vi "Configure Trace.vi"(6 "Trace Unit (0: DBM)":i32(ring) items=["DBM", "W"], 7 "Enable Trace (T: Enable)":bool=TRUE, 8 "error in (no error)":errorcluster, 9 "Trace Duration (0.0001 s)":dbl=0.0001, 10 "Trace Delay (0 s)":dbl, 11 "VISA resource name":refnum<visa-resource-name>) -> (0 "error out":errorcluster, 3 "VISA resource name out":refnum<visa-resource-name>)   [LabVIEW 2014, in "Agilent U2000 Series.lvlib"]
doc: "Configures the measured power trace which includes:\nSpecifying the resolution type of trace to be captured.\nEnables/disables trace capture.\nSpecifying the trace units.\nSetting the duration of the trace and the delay between the delayed trigger point and the start of the trace.\n\nUsing this VI will set the sensor to normal mode. \n\nNotes:\nIn case of U2040 X-Series, it is applicable for U2042XA/U2044XA/U2049XA only."
uses:
  Agilent U2000 Series.lvlib
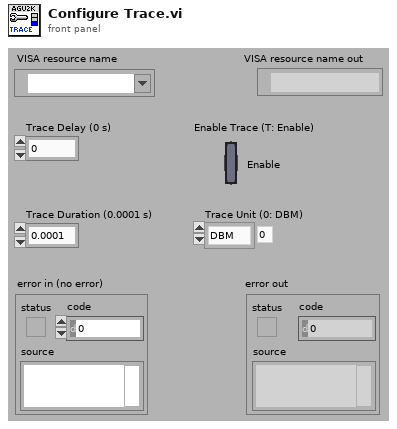
[diagram p1: front panel]
types:
  T1 = typedef "Agilent U2000 Series.lvlib/Extended User Data.ctl" = cluster{"U2000 Series Mode":u16, "Trigger Source Int/Ext":bool}
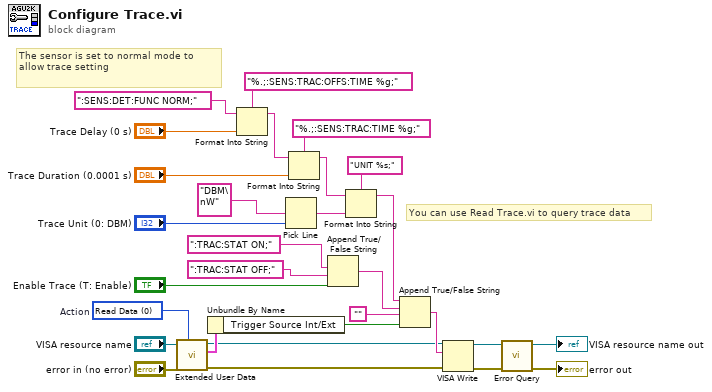
[diagram p0: block diagram]
diagram:
  w7 = 0 items=["Read Data", "Write Data", "Clear Data", "Clear ALL Data"]  # Action
  # "The sensor is set to normal mode to allow trace setting"
  # "You can use Read Trace.vi to query trace data"
  n1 = call "Extended User Data.vi"("Action (1: Write Data)"=w7, "error in (no error)"="error in (no error)", "VISA resource name"="VISA resource name") -> ("error out"=w1:errorcluster, "User Data Out"=w6:T1, "VISA resource name out"=w2:refnum<visa-resource-name>)  [unwired: 1 in, 5 out]
  n2 = Unbundle By Name(w6) -> ("Trigger Source Int/Ext"=w5:bool)
  n3 = Format Into String(format string="%.;:SENS:TRAC:OFFS:TIME %g;", initial string=":SENS:DET:FUNC NORM;", "Trace Delay (0 s)") -> (resulting string=w27:string)  [unwired: 1 in, 1 out]
  n4 = Pick Line(multi-line string="DBM\nW", line index="Trace Unit (0: DBM)") -> (output string=w18:string)  [unwired: 1 out]
  n5 = Format Into String(format string="%.;:SENS:TRAC:TIME %g;", initial string=w27, "Trace Duration (0.0001 s)") -> (resulting string=w24:string)  [unwired: 1 in, 1 out]
  n6 = Append True/False String(1:"Enable Trace (T: Enable)", 2:":TRAC:STAT OFF;", 3:":TRAC:STAT ON;") -> (0:w11:string)  [unwired: 1 out]
  n7 = Format Into String(format string="UNIT %s;", initial string=w24, w18) -> (resulting string=w9:string)  [unwired: 1 in, 1 out]
  n8 = Append True/False String(1:w5, 2:"", 3:w11, 4:w9) -> (0:w8:string)
  n9 = VISA Write(VISA resource name=w2, write buffer=w8, error in (no error)=w1) -> (VISA resource name out=w15:refnum<visa-resource-name>, error out=w16:errorcluster)  [unwired: 1 out]
  n10 = call "Error Query.vi"("error in (no error)"=w16, "VISA resource name"=w15) -> ("error out"=→"error out":errorcluster, "VISA resource name out"=→"VISA resource name out":refnum<visa-resource-name>)  [unwired: 8 out]
